vi "OP500ZP_Test_DataDyn.vi"(4 "Vcell Max (V)":dbl, 5 "MCU":bool, 6 "Vcell Min (V)":dbl, 7 "appdir":path, 8 "errin":errorcluster, 9 "Température usine (°C)":dbl, 10 "Tcell Max (°C)":dbl, 11 "Tcell Min (°C)":dbl) -> (0 "errout":errorcluster, 1 "StrData":T1, 2 "datalog":string, 3 "pass":bool)   [LabVIEW 2020]
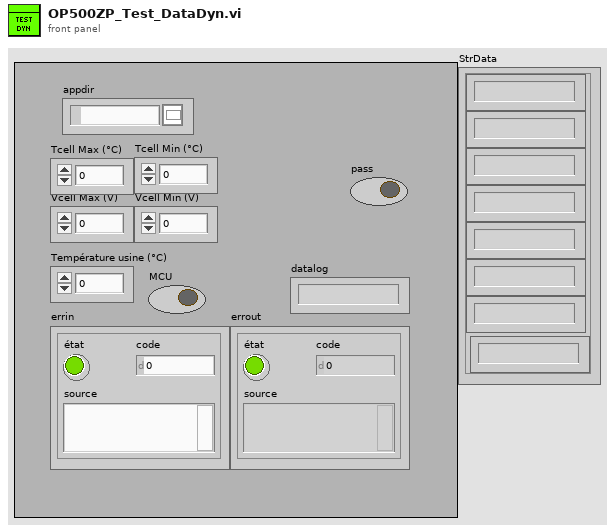
[diagram p1: front panel]
types:
  T1 = cluster{"Chaîne":string, "Chaîne":string, "Chaîne":string, "Chaîne":string, "Chaîne":string, "Chaîne":string, "Chaîne":string, "Chaîne 2":string}
  T2 = cluster{string, string, string, string, string, string, string, "cas vrai":string}
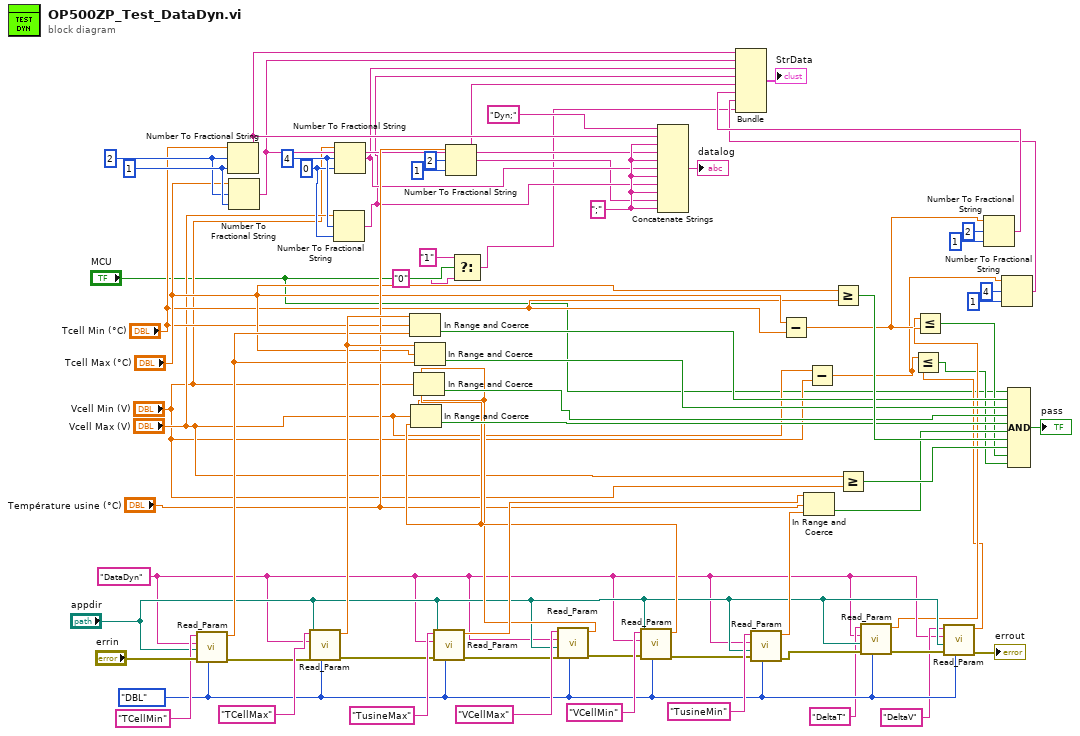
[diagram p0: block diagram]
diagram:
  w36 = ";" ("chaîne")
  w40 = i16 0 ("précision (6)")
  w41 = i16 4 ("largeur (-)")
  w43 = i16 1 ("précision (6)")
  w42 = i16 2 ("largeur (-)")
  w26 = enum16{"STR", "DBL", "U32"}."DBL" ("Énum")
  w22 = "DataDyn" ("section")
  n1 = call <userlib>:"Read_Param.vi"("Énum"=w26, "errin"="errin", 9:"appdir", "section"=w22, "key"="TCellMin") -> ("error out"=w45:errorcluster, "dbl"=w51:dbl)  [unwired: 2 in, 3 out]
  n2 = Number To Fractional String(number="Tcell Min (°C)", width (-)=w42, precision (6)=w43) -> (F-format string=w34:string)  [unwired: 1 in]
  n3 = Number To Fractional String(number="Tcell Max (°C)", width (-)=w42, precision (6)=w43) -> (F-format string=w33:string)  [unwired: 1 in]
  n4 = call <userlib>:"Read_Param.vi"("Énum"=w26, "errin"=w45, 9:"appdir", "section"=w22, "key"="TCellMax") -> ("error out"=w46:errorcluster, "dbl"=w53:dbl)  [unwired: 2 in, 3 out]
  n5 = Number To Fractional String(number="Vcell Max (V)", width (-)=w41, precision (6)=w40) -> (F-format string=w31:string)  [unwired: 1 in]
  n6 = Number To Fractional String(number="Vcell Min (V)", width (-)=w41, precision (6)=w40) -> (F-format string=w32:string)  [unwired: 1 in]
  n7 = In Range and Coerce(upper limit=w53, x="Tcell Min (°C)", lower limit=w51) -> (In Range?=w62:bool)  [unwired: 1 out]
  n8 = In Range and Coerce(upper limit=w53, x="Tcell Max (°C)", lower limit=w51) -> (In Range?=w63:bool)  [unwired: 1 out]
  n9 = call <userlib>:"Read_Param.vi"("Énum"=w26, "errin"=w46, 9:"appdir", "section"=w22, "key"="TusineMax") -> ("error out"=w47:errorcluster, "dbl"=w58:dbl)  [unwired: 2 in, 3 out]
  n10 = Number To Fractional String(number="Température usine (°C)", width (-)=i16 2 ("largeur (-)"), precision (6)=i16 1 ("précision (6)")) -> (F-format string=w30:string)  [unwired: 1 in]
  n11 = Select(t="1" ("cas vrai"), s="MCU", f="0") -> (s? t:f=w1:string)
  n12 = call <userlib>:"Read_Param.vi"("Énum"=w26, "errin"=w47, 9:"appdir", "section"=w22, "key"="VCellMax") -> ("error out"=w48:errorcluster, "dbl"=w55:dbl)  [unwired: 2 in, 3 out]
  n13 = call <userlib>:"Read_Param.vi"("Énum"=w26, "errin"=w48, 9:"appdir", "section"=w22, "key"="VCellMin") -> ("error out"=w49:errorcluster, "dbl"=w56:dbl)  [unwired: 2 in, 3 out]
  n14 = In Range and Coerce(upper limit=w55, x="Vcell Max (V)", lower limit=w56) -> (In Range?=w65:bool)  [unwired: 1 out]
  n15 = In Range and Coerce(upper limit=w55, x="Vcell Min (V)", lower limit=w56) -> (In Range?=w64:bool)  [unwired: 1 out]
  n16 = Concatenate Strings("Dyn;" ("chaîne"), w34, w36, w33, w36, w32, w36, w31, w36, w30, w36) -> (→"datalog":string)
  n17 = call <userlib>:"Read_Param.vi"("Énum"=w26, "errin"=w49, 9:"appdir", "section"=w22, "key"="TusineMin") -> ("error out"=w29:errorcluster, "dbl"=w59:dbl)  [unwired: 2 in, 3 out]
  n18 = Subtract(x="Tcell Max (°C)", y="Tcell Min (°C)") -> (x-y=w9:dbl)
  n19 = In Range and Coerce(upper limit=w58, x="Température usine (°C)", lower limit=w59) -> (In Range?=w66:bool)  [unwired: 1 out]
  n20 = Subtract(x="Vcell Max (V)", y="Vcell Min (V)") -> (x-y=w6:dbl)
  n21 = Greater Or Equal?(x="Tcell Max (°C)", y="Tcell Min (°C)") -> (x >= y?=w67:bool)
  n22 = Greater Or Equal?(x="Vcell Max (V)", y="Vcell Min (V)") -> (x >= y?=w68:bool)
  n23 = call <userlib>:"Read_Param.vi"("Énum"=w26, "errin"=w29, 9:"appdir", "section"=w22, "key"="DeltaT") -> ("error out"=w28:errorcluster, "dbl"=w17:dbl)  [unwired: 2 in, 3 out]
  n24 = Less Or Equal?(x=w9, y=w17) -> (x <= y?=w15:bool)
  n25 = call <userlib>:"Read_Param.vi"("Énum"=w26, "errin"=w28, 9:"appdir", "section"=w22, "key"="DeltaV") -> ("error out"=→"errout":errorcluster, "dbl"=w16:dbl)  [unwired: 2 in, 3 out]
  n26 = Less Or Equal?(x=w6, y=w16) -> (x <= y?=w14:bool)
  n27 = Number To Fractional String(number=w9, width (-)=i16 2 ("largeur (-)"), precision (6)=i16 1 ("précision (6)")) -> (F-format string=w8:string)  [unwired: 1 in]
  n28 = Number To Fractional String(number=w6, width (-)=i16 4 ("largeur (-)"), precision (6)=i16 1 ("précision (6)")) -> (F-format string=w7:string)  [unwired: 1 in]
  n29 = Bundle(w34, w33, w32, w31, w30, w8, w7, "cas vrai"=w1) -> (→"StrData":T2)  [unwired: 1 in]
  n30 = Compound Arithmetic op=AND ("Opérateur arithmétique")("MCU", w62, w63, w64, w65, w66, w67, w68, w15, w14) -> (→"pass":bool)
